vi "V7310.Main.Select.vi"(8 "error in":errorcluster, 10 "Job":string, 11 "Data in":T1={"Status"={"State"=enum."Init", "LaserStatus"=enum."-", "LaserStatusRaw"="", "Ref"=refnum, "RTC TS"=timestamp(0 s since 1904-01-01), "Conn TS"=timestamp(0 s since 1904-01-01), "Msg"=[], "JobInUse"="", "Jobs"=[], "Vars"=[]}, "Sets"={"Address"="192.168.2.1", "Timeout_ms"=5000, "ReconnectPeriod_s"=0, "JobInUse"="", "CoordinatesOffset"={"X"=0.0, "Y"=0.0}}}) -> (0 "error out":errorcluster, 3 "Data out":T1={"Status"={"State"=enum."Init", "LaserStatus"=enum."-", "LaserStatusRaw"="", "Ref"=refnum, "RTC TS"=timestamp(0 s since 1904-01-01), "Conn TS"=timestamp(0 s since 1904-01-01), "Msg"=[], "JobInUse"="", "Jobs"=[], "Vars"=[]}, "Sets"={"Address"="192.168.2.1", "Timeout_ms"=5000, "ReconnectPeriod_s"=0, "JobInUse"="", "CoordinatesOffset"={"X"=0.0, "Y"=0.0}}})   [LabVIEW 2015]
uses:
  V7310.Data.ctl
  V7310.Data.Status.ctl
  V7310.Data.Status.State.ctl
  LowLevel/V7310.LaserStatus.ctl
  LowLevel/V7310.Message.Data.ctl
  LowLevel/V7310.Job.Variable.ctl
  V7310.Data.Sets.ctl
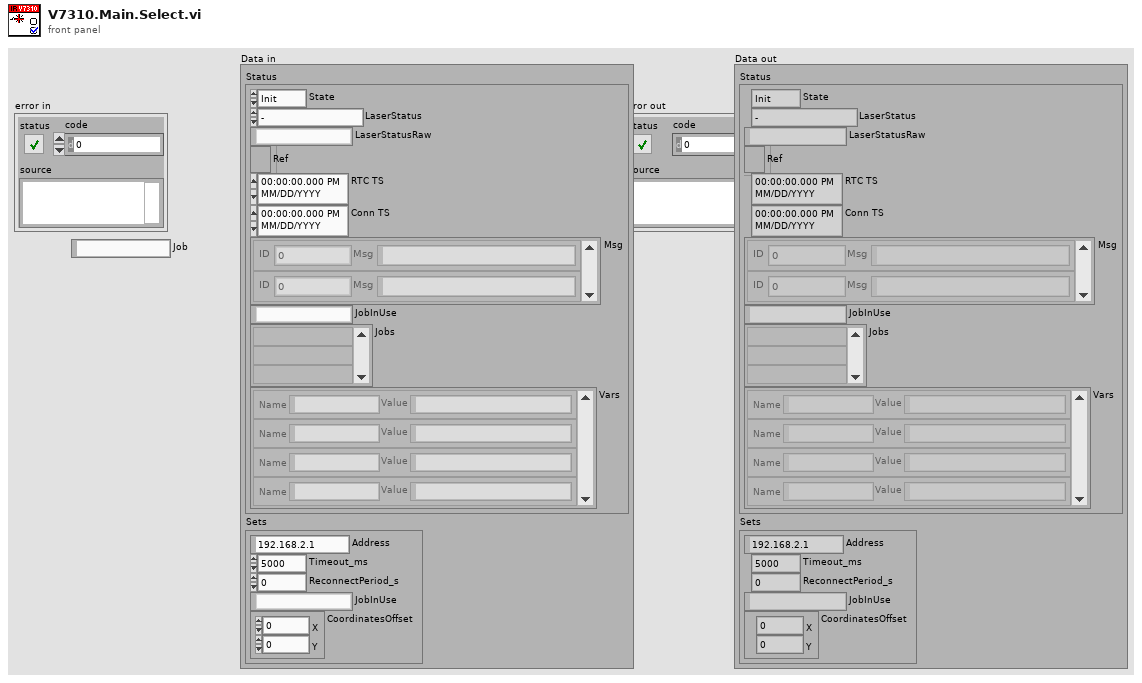
[diagram p1: front panel]
types:
  T1 = typedef "V7310.Data.ctl" = cluster{"Status":T2, "Sets":T7}
  T2 = typedef "V7310.Data.Status.ctl" = cluster{"State":T3, "LaserStatus":T4, "LaserStatusRaw":string, "Ref":refnum<k5>, "RTC TS":timestamp, "Conn TS":timestamp, "Msg":T5[], "JobInUse":string, "Jobs":string[], "Vars":T6[]}
  T3 = typedef "V7310.Data.Status.State.ctl" = enum16{"First", "Init", "Msg", "Error", "Abort", "Idle", "Run"}
  T4 = typedef "V7310.LaserStatus.ctl" = enum16{"-", "Initialize", "KeySwitchOpen", "TimeoutInterlock", "InterlockOpen", "StartUp", "ShutterlockOpen", "Standby", "Ready", "PrepareForMarking", "WaitForTrigger", "Marking"}
  T5 = typedef "V7310.Message.Data.ctl" = cluster{"ID":i32, "Msg":string}
  T6 = typedef "V7310.Job.Variable.ctl" = cluster{"Name":string, "Value":string}
  T7 = typedef "V7310.Data.Sets.ctl" = cluster{"Address":string, "Timeout_ms":i32, "ReconnectPeriod_s":i32, "JobInUse":string, "CoordinatesOffset":cluster{"X":dbl, "Y":dbl}}
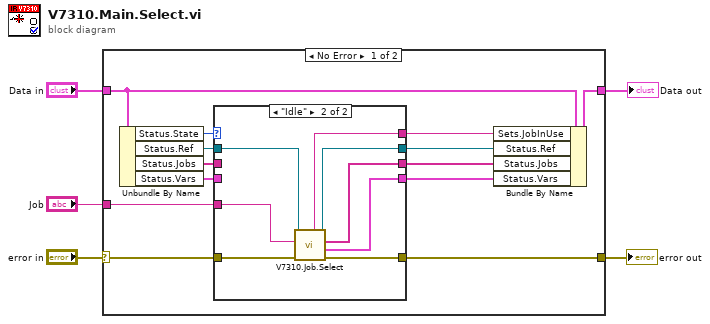
[diagram p0: block diagram]
diagram:
  n1 = case shown="No Error" "error in" {
    selector: "error in" -> [w14 w33]
    tunnel: [w13 w33] -> w4
    tunnel: "Data in" -> [w17 w32]
    tunnel: [w18 w32] -> w2
    tunnel: "Job" -> [w11 _]
    frame No Error {
      n2 = Unbundle By Name(w17) -> ("Status.State"=w10:T3, "Status.Ref"=w15:refnum<k5>, "Status.Jobs"=w7:string[], "Status.Vars"=w6:T6[])
      n3 = case shown="\"Idle\"" w10 {
        tunnel: [w23 w31] -> w13
        tunnel: [w22 w30] -> w16
        tunnel: w15 -> [w22 w29]
        tunnel: w14 -> [w23 w28]
        tunnel: [w21 w26] -> w12
        tunnel: w11 -> [w21 w27]
        tunnel: [w20 w25] -> w9
        tunnel: [w19 w24] -> w8
        tunnel: w7 -> [w20 _]
        tunnel: w6 -> [w19 _]
        frame Default {
        }
        frame "Idle" {
          n4 = call "V7310.Job.Select.vi"("error in"=w28, "Job"=w27, "Connection in"=w29) -> ("error out"=w31:errorcluster, "VarNames"=w24:T6[], "Jobs"=w25:string[], "Connection out"=w30:refnum<k5>, "Selected Job"=w26:string)  [unwired: 4 in]
        }
      }
      n5 = Bundle By Name(cluster=w17, "Sets.JobInUse"=w12, "Status.Ref"=w16, "Status.Jobs"=w9, "Status.Vars"=w8) -> (w18:T1)
    }
    frame Error {
    }
  }
  "error out" <- w4
  "Data out" <- w2
